vi "3.1-Lidar Angle Setpoint Calibration.vi"(1 "mph":i32) -> (0 "setpoint":i32)   [LabVIEW 2010]
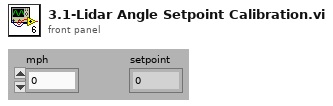
[diagram p1: front panel]
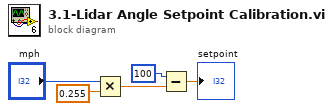
[diagram p0: block diagram]
diagram:
  n1 = Multiply(x="mph", y=0.255) -> (x*y=w4:dbl)
  n2 = Subtract(x=100 ("mph"), y=w4) -> (x-y=→"setpoint":dbl)
